vi "8P_EnFlo_Specific.vi"(4 "Datalog file path (full)":path, 5 "COM port":refnum<visa-resource-name>, 6 "Log data stream":bool, 7 "Data rate (Hz)":u8(ring)=14 items=["1", "2", "4", "5", "8", "10", "16", "20", "25", "32", "40", "50", "64", "80", "100", "125", "160", "200", "250", "320", "400", "500", "625", "800", "1000"], 8 "N samples":u32=1000, 9 "Command":T2="s") -> (0 "Output Freq Hz":dbl, 1 "Error":errorcluster, 2 "All samples out":sgl[][](array[numeric]), 3 "Rendezvous Out":bool)   [LabVIEW 2020]
uses:
  ctls/Cmd.ctl
  <vilib>/Analysis/baseanly.llb/Mean (DBL).vi
  <vilib>/Analysis/NI_AALBase.lvlib
  Globals/Meas_global.vi
panel:
  in  "Main":T1(tab)
  out "Pressure sensor EEPROM checksums ok":bool[](array[boolean])
  out "Pressure sensor temperatures in range":bool[](array[boolean])
  out "Pressure sensor values in range":bool[](array[boolean])
  out "Subsystems ok":bool[](array[boolean])
  out "P_raw_Azero":sgl[](array[numeric])
  out "n":u16
  out "Auto zero progBar":u16(slide) caption="Collecting samples, please maintain dP = 0" scale=0.0..1000.0
  out "Chk ok":bool
  out "EEPROM Checksum":u8 format="%02x"
  in  "EEPROM array":sgl[](array[numeric])
  out "No of Samples Requested":u32
  out "No of Samples Acquired":i32
  out "Downsampling (N)":i32
  out "Acquisiton Freq Hz":dbl
  out "sent":bool
  in  "Stop Data":bool
  out "External thermistor temperature (°C)":sgl
  out "Checksum ok":bool
  out "Pressures":sgl[][](graph)
  out "Stream enabled":bool
  out "frm err":u32
  out "chk err":u32
  # "Paul Nathan 08/2017"
  # "Output array order:\nP0......... (Pa)\n.\n.\nP7......... (Pa)\nT_ext.... (deg C)\nT0..........(deg C)\n.\n.\nT7......... (deg C)"
  # "External thermistor value in range"
  # "MCU EEPROM checksum ok"
  # "Pressure sensor 0 EEPROM checksum okay"
  # "Pressure sensor 1 EEPROM checksum okay"
  # "Pressure sensor 2 EEPROM checksum okay"
  # "Pressure sensor 3 EEPROM checksum okay"
  # "Pressure sensor 4 EEPROM checksum okay"
  # "Pressure sensor 5 EEPROM checksum okay"
  # "Pressure sensor 6 EEPROM checksum okay"
  # "Pressure sensor 0 temperature in range"
  # "Pressure sensor 1 temperature in range"
  # "Pressure sensor 2 temperature in range"
  # "Pressure sensor 3 temperature in range"
  # "Pressure sensor 4 temperature in range"
  # "Pressure sensor 5 temperature in range"
  # "Pressure sensor 6 temperature in range"
  # "Pressure sensor 0 value in range"
  # "Pressure sensor 1 value in range"
  # "Pressure sensor 2 value in range"
  # "Pressure sensor 3 value in range"
  # "Pressure sensor 4 value in range"
  # "Pressure sensor 5 value in range"
  # "Pressure sensor 6 value in range"
  # "of 1000"
  # "P0 raw auto-zero"
  # "P1 raw auto-zero"
  # "P2 raw auto-zero"
  # "P3 raw auto-zero"
  # "P4 raw auto-zero"
  # "P5 raw auto-zero"
  # "P6 raw auto-zero"
  # "P7 raw auto-zero"
  # "P0 raw auto-zero"
  # "P1 raw auto-zero"
  # "P2 raw auto-zero"
  # "P3 raw auto-zero"
  # "P4 raw auto-zero"
  # "P5 raw auto-zero"
  # "P6 raw auto-zero"
  # "P7 raw auto-zero"
  # "External thermistor temperature offset (deg C)"
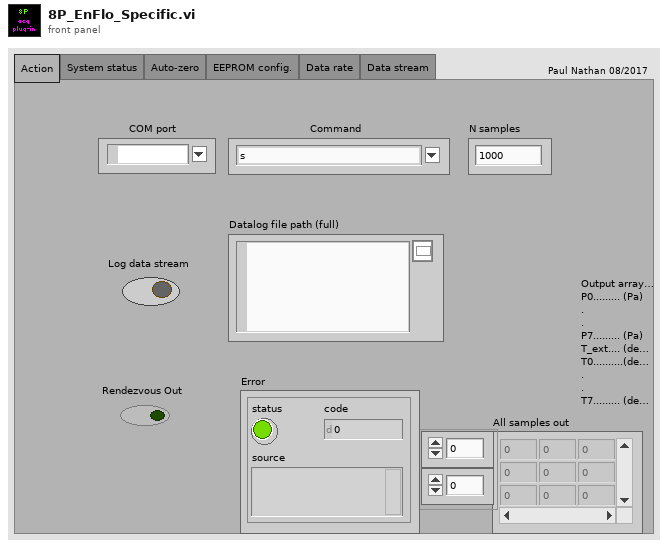
[diagram p1: front panel]
types:
  T1 = enum32{"Action", "System status", "Auto-zero", "EEPROM config.", "Data rate", "Data stream"}
  T2 = typedef "Cmd.ctl" = string
  T3 = enum16{"open", "replace", "create", "open or create", "replace or create", "replace or create with confirmation"}
  T4 = typedef "Rendezvous RefNum" = refnum<k1>
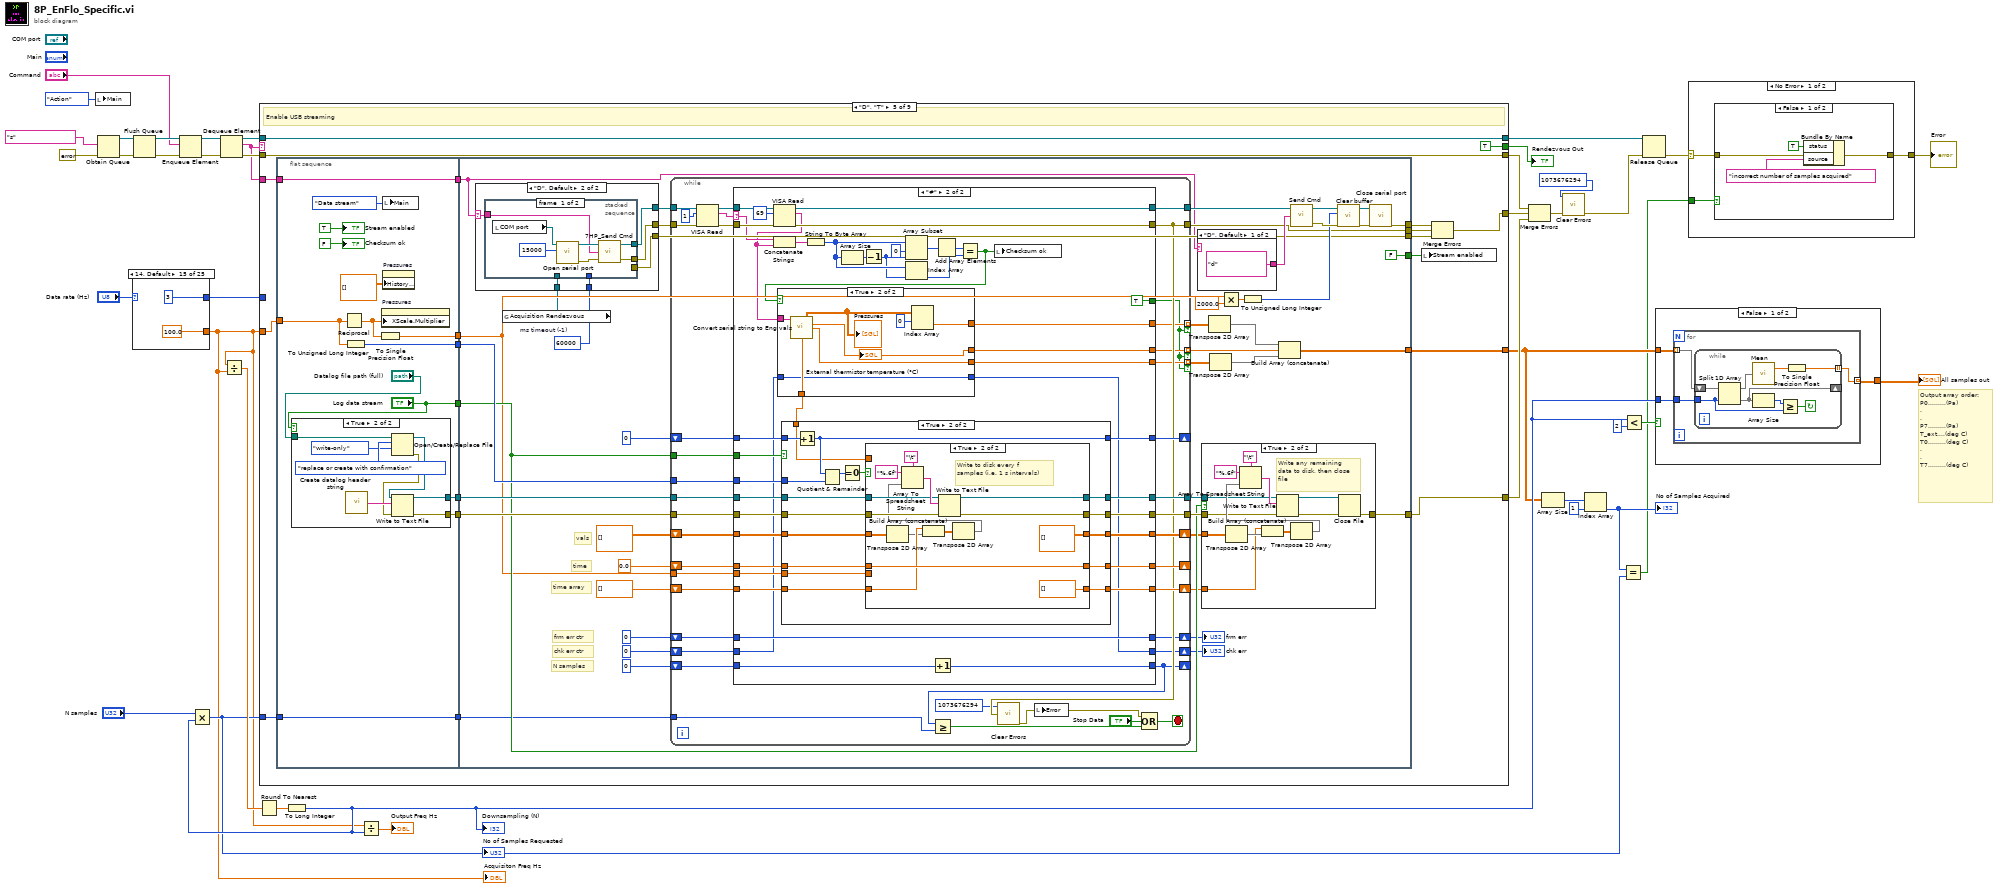
[diagram p0: block diagram]
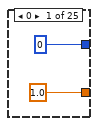
[diagram p5: hidden frame]
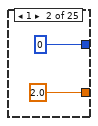
[diagram p6: hidden frame]
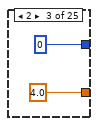
[diagram p7: hidden frame]
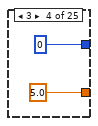
[diagram p8: hidden frame]
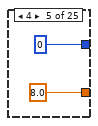
[diagram p9: hidden frame]
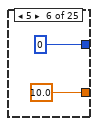
[diagram p10: hidden frame]
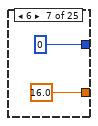
[diagram p11: hidden frame]
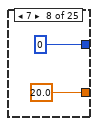
[diagram p12: hidden frame]
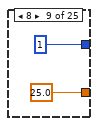
[diagram p13: hidden frame]
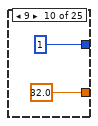
[diagram p14: hidden frame]
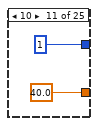
[diagram p15: hidden frame]
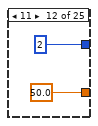
[diagram p16: hidden frame]
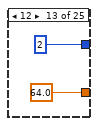
[diagram p17: hidden frame]
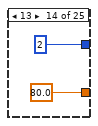
[diagram p18: hidden frame]
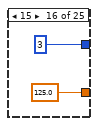
[diagram p19: hidden frame]
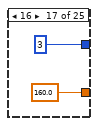
[diagram p20: hidden frame]
diagram:
  # "Output array order:\nP0.........(Pa)\n.\n.\nP7.........(Pa)\nT_ext....(deg C)\nT0.........(deg C)\n.\n.\nT7.........(deg C)"
  n1 = local write "Main"(T1."Action" ("Main")) -> ()
  n2 = Obtain Queue(element data type=T2 "s" ("Combo Box"), error in (no error)=errorcluster {"status"=FALSE, "code"=0, "source"=""}) -> (queue out=w38:refnum<queue>, error out=w39:errorcluster)  [unwired: 3 in, 1 out]
  n3 = case shown="14, Default" "Data rate (Hz)" {
    tunnel: [1.0 2.0 4.0 5.0 8.0 10.0 16.0 20.0 25.0 32.0 40.0 50.0 64.0 80.0 100.0 125.0 160.0 200.0 250.0 320.0 400.0 500.0 625.0 800.0 1000.0] -> w2
    tunnel: [u8 0 u8 0 u8 0 u8 0 u8 0 u8 0 u8 0 u8 0 u8 1 u8 1 u8 1 u8 2 u8 2 u8 2 u8 3 u8 3 u8 3 u8 4 u8 4 u8 4 u8 5 u8 5 u8 6 u8 6 u8 6] -> w1
    frame 0 {
    }
    frame 1 {
    }
    frame 2 {
    }
    frame 3 {
    }
    frame 4 {
    }
    frame 5 {
    }
    frame 6 {
    }
    frame 7 {
    }
    frame 8 {
    }
    frame 9 {
    }
    frame 10 {
    }
    frame 11 {
    }
    frame 12 {
    }
    frame 13 {
    }
    frame 14, Default {
    }
    frame 15 {
    }
    frame 16 {
    }
    frame 17 {
    }
    frame 18 {
    }
    frame 19 {
    }
    frame 20 {
    }
    frame 21 {
    }
    frame 22 {
    }
    frame 23 {
    }
    frame 24 {
    }
  }
  "Acquisiton Freq Hz" <- w2
  n4 = Flush Queue(queue=w38, error in (no error)=w39) -> (queue out=w37:refnum<queue>, error out=w33:errorcluster)  [unwired: 1 out]
  n5 = Enqueue Element(queue=w37, element="Command", error in (no error)=w33) -> (queue out=w34:refnum<queue>, error out=w32:errorcluster)  [unwired: 1 in, 1 out]
  n6 = Dequeue Element(queue=w34, error in (no error)=w32) -> (queue out=w29:refnum<queue>, element=w27:T2, error out=w28:errorcluster)  [unwired: 1 in, 1 out]
  n7 = Divide(x=w2, y=w2) -> (x/y=w17:dbl)
  n8 = Round To Nearest(number=w17) -> (nearest integer value=w16:dbl)
  n9 = To Long Integer(number=w16) -> (32bit integer=w12:i32)
  "Downsampling (N)" <- w12
  n10 = Multiply(x="N samples", y=w12) -> (x*y=w4:u32)
  "No of Samples Requested" <- w4
  n11 = case shown="\"D\", \"T\"" w27 {
    tunnel: w29 -> [w96 w135 w172 w213 w265 w544 w574 w601 w605]
    tunnel: [w96 w135 w172 w213 w265 w544 w574 w601 w605] -> w30
    tunnel: w28 -> [w95 w134 w171 w212 w264 w543 w575 w600 w604]
    tunnel: [w95 w134 w171 w212 w264 w543 w575 w600 w604] -> w26
    tunnel: w27 -> [w94 w133 w170 w211 w263 w546 w572 _ _]
    tunnel: [w92 w131 w168 w208 w248 w545 w570 errorcluster {"status"=FALSE, "code"=0, "source"=""} ("Error out") errorcluster {"status"=FALSE, "code"=0, "source"=""} ("Error out")] -> w25
    tunnel: [_ _ _ _ w261 _ _ _ _] -> w24
    tunnel: w2 -> [_ _ _ _ w257 w542 w568 _ _]
    tunnel: w4 -> [_ _ _ _ w253 _ _ _ _]
    tunnel: [_ _ _ _ w251 _ _ _ _] -> w11
    tunnel: [FALSE FALSE FALSE FALSE TRUE FALSE FALSE FALSE FALSE] -> w3
    tunnel: w1 -> [_ _ _ _ _ _ w567 _ _]
    frame "S", "s" {
      # "Perform self-test and retrieve status bytes, Retrieve status bytes"
      n12 = flat-sequence {
        tunnel: w94 -> [w99]
        tunnel: [w99] -> w93
        tunnel: w93 -> [w105]
        tunnel: [w100] -> w92
        frame #0 {
          w98 = bool[] [] ("Pressure sensor EEPROM checksums ok")
          n13 = local write "Main"(T1."System status" ("Main")) -> ()
          "Pressure sensor EEPROM checksums ok" <- w98
          "Pressure sensor temperatures in range" <- w98
          "Pressure sensor values in range" <- w98
          "Subsystems ok" <- w98
        }
        frame #1 {
          w109 = 1 ("length (rest)")
          w117 = u8 0 ("byte count")
          n14 = local read "COM port"() -> (w106:refnum<visa-resource-name>)
          n15 = call "Open serial port.vi"("timeout (ms)"=u32 5000, "VISA resource name"=w106) -> ("Error out"=w127:errorcluster, "VISA resource name out"=w128:refnum<visa-resource-name>)  [unwired: 8 in]
          n16 = call "Send Cmd.vi"("Error In"=w127, "Operation"=w105, "Port"=w128) -> ("Error Out"=w125:errorcluster, "Port out"=w126:refnum<visa-resource-name>)  [unwired: 1 in]
          n17 = VISA Read(VISA resource name=w126, byte count=u32 4, error in (no error)=w125) -> (VISA resource name out=w123:refnum<visa-resource-name>, read buffer=w112:string, error out=w122:errorcluster)  [unwired: 1 out]
          n18 = call "Close serial port.vi"("Error in"=w122, "VISA resource name"=w123) -> ("Error out"=w100:errorcluster)  [unwired: 9 in]
          n19 = String Subset(string=w112, offset (0)=0, length (rest)=w109) -> (substring=w121:string)
          n20 = String Subset(string=w112, offset (0)=1, length (rest)=w109) -> (substring=w120:string)
          n21 = String Subset(string=w112, offset (0)=2 ("length (rest)"), length (rest)=w109) -> (substring=w119:string)
          n22 = String Subset(string=w112, offset (0)=3, length (rest)=w109) -> (substring=w118:string)
          n23 = Type Cast(type=w117, x=w121) -> (*(type *) &x=w116:u8)
          n24 = Type Cast(type=w117, x=w120) -> (*(type *) &x=w115:u8)
          n25 = Type Cast(type=w117, x=w119) -> (*(type *) &x=w114:u8)
          n26 = Type Cast(type=w117, x=w118) -> (*(type *) &x=w113:u8)
          n27 = Number To Boolean Array(number=w116) -> (Boolean array=w104:bool[])
          n28 = Number To Boolean Array(number=w115) -> (Boolean array=w103:bool[])
          n29 = Number To Boolean Array(number=w114) -> (Boolean array=w102:bool[])
          n30 = Number To Boolean Array(number=w113) -> (Boolean array=w101:bool[])
          n31 = local write "Pressure sensor EEPROM checksums ok"(w104) -> ()
          n32 = local write "Pressure sensor temperatures in range"(w103) -> ()
          n33 = local write "Pressure sensor values in range"(w102) -> ()
          n34 = local write "Subsystems ok"(w101) -> ()
        }
      }
    }
    frame "Z", "z" {
      # "Perform permanent auto-zero (write values to EEPROM), Perform temporary auto-zero"
      n35 = flat-sequence {
        tunnel: w133 -> [w139]
        tunnel: [w139] -> w132
        tunnel: w132 -> [w146]
        tunnel: [w142] -> w131
        frame #0 {
          n36 = local write "Main"(T1."Auto-zero" ("Main")) -> ()
          "P_raw_Azero" <- sgl[] [] ("P_raw_Azero")
          "Auto zero progBar" <- u16 0 ("Collecting samples, please maintain dP = 0")
        }
        frame #1 {
          n37 = local read "COM port"() -> (w147:refnum<visa-resource-name>)
          n38 = call "Open serial port.vi"("timeout (ms)"=u32 16000, "VISA resource name"=w147) -> ("Error out"=w153:errorcluster, "VISA resource name out"=w154:refnum<visa-resource-name>)  [unwired: 8 in]
          n39 = call "Send Cmd.vi"("Error In"=w153, "Operation"=w146, "Port"=w154) -> ("Error Out"=w151:errorcluster, "Port out"=w152:refnum<visa-resource-name>)  [unwired: 1 in]
          n40 = VISA Read(VISA resource name=w152, byte count=u32 32, error in (no error)=w151) -> (VISA resource name out=w149:refnum<visa-resource-name>, read buffer=w143:string, error out=w148:errorcluster)  [unwired: 1 out]
          n41 = for {
            N: 1000 -> [_]
            shift-right: [w156] -> _
            shift-left: u16 0 -> [w157]
            n42 = Increment(x=w157) -> (x+1=w156:u16)
            "n" <- w156
            n43 = Wait (ms)(milliseconds to wait=u32 11) -> ()  [unwired: 1 out]
            n44 = local write "Auto zero progBar"(w156) -> ()
          }
          n45 = for {
            N: 8 -> [_]
            tunnel: [w160] -> w145 mode=indexing
            tunnel: w143 -> [w159]
            i -> [w166]
            w164 = 4 ("x")
            # "to BE"
            n46 = Multiply(x=w164, y=w166) -> (x*y=w165:i32)
            n47 = String Subset(string=w159, offset (0)=w165, length (rest)=w164) -> (substring=w163:string)
            n48 = Reverse String(1:w163) -> (0:w162:string)
            n49 = Type Cast(type=sgl 0.0 ("byte count"), x=w162) -> (*(type *) &x=w160:sgl)
          }
          n50 = call "Close serial port.vi"("Error in"=w148, "VISA resource name"=w149) -> ("Error out"=w142:errorcluster)  [unwired: 9 in]
          n51 = local write "P_raw_Azero"(w145) -> ()
        }
      }
    }
    frame "R" {
      # "Read all EEPROM values"
      n52 = flat-sequence {
        tunnel: w170 -> [w175]
        tunnel: [w175] -> w169
        tunnel: w169 -> [w189]
        tunnel: [w176] -> w168
        frame #0 {
          n53 = local write "EEPROM array"(sgl[] [] ("EEPROM array")) -> ()
          n54 = local write "Main"(T1."EEPROM config." ("Main")) -> ()
        }
        frame #1 {
          n55 = local read "COM port"() -> (w190:refnum<visa-resource-name>)
          n56 = call "Open serial port.vi"("timeout (ms)"=u32 5000, "VISA resource name"=w190) -> ("Error out"=w196:errorcluster, "VISA resource name out"=w197:refnum<visa-resource-name>)  [unwired: 8 in]
          n57 = call "Send Cmd.vi"("Error In"=w196, "Operation"=w189, "Port"=w197) -> ("Error Out"=w194:errorcluster, "Port out"=w195:refnum<visa-resource-name>)  [unwired: 1 in]
          n58 = VISA Read(VISA resource name=w195, byte count=u32 37, error in (no error)=w194) -> (VISA resource name out=w192:refnum<visa-resource-name>, read buffer=w185:string, error out=w191:errorcluster)  [unwired: 1 out]
          n59 = String To Byte Array(string=w185) -> (unsigned byte array=w179:u8[])
          n60 = call "Close serial port.vi"("Error in"=w191, "VISA resource name"=w192) -> ("Error out"=w176:errorcluster)  [unwired: 9 in]
          n61 = for {
            N: 9 -> [_]
            tunnel: [w202] -> w187 mode=indexing
            tunnel: w185 -> [w201]
            i -> [w206]
            w204 = 4 ("x")
            # "to BE"
            n62 = Multiply(x=w204, y=w206) -> (x*y=w205:i32)
            n63 = String Subset(string=w201, offset (0)=w205, length (rest)=w204) -> (substring=w200:string)
            n64 = Reverse String(1:w200) -> (0:w199:string)
            n65 = Type Cast(type=sgl 0.0 ("byte count"), x=w199) -> (*(type *) &x=w202:sgl)
          }
          n66 = Array Size(array=w179) -> (size(s)=w181:i32)
          n67 = Decrement(x=w181) -> (x-1=w180:i32)
          n68 = Index Array(array=w179, index=36) -> (element=w183:u8)
          n69 = Array Subset(array=w179, index=0, length=w180) -> (w177:u8[])
          n70 = Add Array Elements(numeric array=w177) -> (sum=w178:u8)
          n71 = Equal?(x=w183, y=w178) -> (x = y?=w186:bool)
          n72 = local write "EEPROM array"(w187) -> ()
          n73 = local write "EEPROM Checksum"(w183) -> ()
          n74 = local write "Chk ok"(w186) -> ()
        }
      }
    }
    frame "W" {
      # "Write all EEPROM values (including new checksum)"
      n75 = flat-sequence {
        tunnel: w211 -> [w216]
        tunnel: [w216] -> w210
        tunnel: ["EEPROM array"] -> w209
        tunnel: w210 -> [w231]
        tunnel: w209 -> [w224]
        tunnel: [w217] -> w208
        frame #0 {
          n76 = local write "Main"(T1."EEPROM config." ("Main")) -> ()
        }
        frame #1 {
          n77 = local read "COM port"() -> (w232:refnum<visa-resource-name>)
          n78 = call "Open serial port.vi"("timeout (ms)"=u32 5000, "VISA resource name"=w232) -> ("Error out"=w237:errorcluster, "VISA resource name out"=w238:refnum<visa-resource-name>)  [unwired: 8 in]
          n79 = call "Send Cmd.vi"("Error In"=w237, "Operation"=w231, "Port"=w238) -> ("Error Out"=w235:errorcluster, "Port out"=w236:refnum<visa-resource-name>)  [unwired: 1 in]
          n80 = for {
            N: 9 -> [_]
            tunnel: w224 -> [w242] mode=indexing
            shift-right: [w243] -> w219
            shift-left: "" -> [w244]
            # "to LE"
            n81 = Type Cast(type="", x=w242) -> (*(type *) &x=w241:string)
            n82 = Reverse String(1:w241) -> (0:w240:string)
            n83 = Concatenate Strings(w244, w240) -> (w243:string)
          }
          n84 = String To Byte Array(string=w219) -> (unsigned byte array=w222:u8[])
          n85 = Array Size(array=w222) -> (size(s)=w220:i32)
          n86 = Array Subset(array=w222, index=0, length=w220) -> (w221:u8[])
          n87 = Add Array Elements(numeric array=w221) -> (sum=w218:u8)
          "EEPROM Checksum" <- w218
          n88 = Type Cast(type="", x=w218) -> (*(type *) &x=w227:string)
          n89 = Concatenate Strings(w219, w227) -> (w226:string)
          n90 = VISA Write(VISA resource name=w236, write buffer=w226, error in (no error)=w235) -> (VISA resource name out=w234:refnum<visa-resource-name>, error out=w233:errorcluster)  [unwired: 1 out]
          n91 = call "Close serial port.vi"("Error in"=w233, "VISA resource name"=w234) -> ("Error out"=w217:errorcluster)  [unwired: 9 in]
          "Chk ok" <- TRUE ("Chk ok")
        }
      }
    }
    frame "D", "T" {
      # "Enable USB streaming"
      n92 = flat-sequence {
        tunnel: w263 -> [w279]
        tunnel: [w279] -> w262
        tunnel: [w276] -> w260
        tunnel: [w275] -> w259
        tunnel: [w273] -> w258
        tunnel: w257 -> [w274]
        tunnel: [w271] -> w256
        tunnel: ["Log data stream"] -> w255
        tunnel: w253 -> [w267]
        tunnel: [w267] -> w252
        tunnel: w262 -> [w292]
        tunnel: [w333] -> w249
        tunnel: [w332] -> w261
        tunnel: w260 -> [w329]
        tunnel: w259 -> [w328]
        tunnel: w258 -> [w330]
        tunnel: w256 -> [w314]
        tunnel: w255 -> [w322]
        tunnel: [FALSE] -> w254
        tunnel: w252 -> [w308]
        tunnel: [w305] -> w251
        tunnel: [w294] -> w247
        tunnel: [w293] -> w246
        frame #0 {
          n93 = case shown="True" "Log data stream" {
            tunnel: "Datalog file path (full)" -> [_ w289]
            tunnel: [refnum<file> refnum ("refnum out") w283] -> w276
            tunnel: [errorcluster {"status"=FALSE, "code"=0, "source"=""} ("error out") w282] -> w275
            frame False {
            }
            frame True {
              n94 = call "Create datalog header string.vi"() -> ("Datalog header string"=w285:string)  [unwired: 1 in]
              n95 = Open/Create/Replace File(file path (use dialog)=w289, operation (0:open)=T3."replace or create with confirmation", access (0:read/write)=enum16{"read/write", "read-only", "write-only"}."write-only") -> (refnum out=w286:refnum<file>, error out=w284:errorcluster)  [unwired: 3 in, 1 out]
              n96 = Write to Text File(file (use dialog)=w286, text=w285, error in=w284) -> (refnum out=w283:refnum<file>, error out=w282:errorcluster)  [unwired: 1 in, 1 out]
            }
          }
          n97 = Reciprocal(x=w274) -> (1/x=w272:dbl)
          n98 = To Unsigned Long Integer(number=w274) -> (unsigned 32bit integer=w273:u32)
          n99 = To Single Precision Float(number=w272) -> (single precision float=w271:sgl)
          n100 = property on="Pressures" class="WFChart (strict)"("XScale.Multiplier"=w272) -> ()  [unwired: 2 in, 2 out]
          n101 = local write "Main"(T1."Data stream" ("Main")) -> ()
          n102 = property on="Pressures" class="WFChart (strict)"("History Data"=sgl[][] []) -> ()  [unwired: 2 in, 2 out]
          "Checksum ok" <- FALSE ("Checksum ok")
          "Stream enabled" <- TRUE ("Stream enabled")
        }
        frame #1 {
          w298 = 60000  # ms timeout (-1)
          # "N samples"
          # "chk err ctr"
          # "frm err ctr"
          # "vals"
          # "time"
          # "time array"
          n103 = global read "Meas_global.vi" "Acquisition Rendezvous"() -> (w297:T4)
          n104 = case shown="\"D\", Default" w292 {
            selector: w292 -> [w339 w355]
            tunnel: [w338 w354] -> w295
            tunnel: [w337 w353] -> w296
            tunnel: [w336 w352] -> w293
            tunnel: w297 -> [w335 w351]
            tunnel: w298 -> [w334 w350]
            frame "T" {
              n105 = stacked-sequence {
                tunnel: w339 -> [w342 _]
                tunnel: [w341 _] -> w338
                tunnel: [w340 _] -> w337
                tunnel: [_ w349] -> w336
                tunnel: w335 -> [_ w348]
                tunnel: w334 -> [_ w347]
                frame #0 {
                  n106 = local read "COM port"() -> (w343:refnum<visa-resource-name>)
                  n107 = call "Open serial port.vi"("timeout (ms)"=u32 15000, "VISA resource name"=w343) -> ("Error out"=w346:errorcluster, "VISA resource name out"=w345:refnum<visa-resource-name>)  [unwired: 8 in]
                  n108 = call "7HP_Send Cmd, wait for ack.vi"("Error In"=w346, "Operation"=w342, "Port"=w345) -> ("Error Out"=w341:errorcluster, "Port out"=w340:refnum<visa-resource-name>)  [unwired: 1 out]
                }
                frame #1 {
                  # "Wait here until all acq. devs. are ready."
                  n109 = call <vilib>:"Wait at Rendezvous.vi"("ms timeout (-1)"=w347, "rendezvous"=w348) -> ("error out"=w349:errorcluster)  [unwired: 3 in, 2 out]
                }
              }
            }
            frame "D", Default {
              n110 = stacked-sequence {
                tunnel: w355 -> [w359 _]
                tunnel: [w356 _] -> w354
                tunnel: [w357 _] -> w353
                tunnel: [_ w365] -> w352
                tunnel: w351 -> [_ w364]
                tunnel: w350 -> [_ w363]
                frame #0 {
                  n111 = local read "COM port"() -> (w361:refnum<visa-resource-name>)
                  n112 = call "Open serial port.vi"("timeout (ms)"=u32 15000, "VISA resource name"=w361) -> ("Error out"=w358:errorcluster, "VISA resource name out"=w360:refnum<visa-resource-name>)  [unwired: 8 in]
                  n113 = call "7HP_Send Cmd.vi"("Error In"=w358, "Operation"=w359, "Port"=w360) -> ("Error Out"=w356:errorcluster, "Port out"=w357:refnum<visa-resource-name>)  [unwired: 1 in]
                }
                frame #1 {
                  # "Wait here until all acq. devs. are ready."
                  n114 = call <vilib>:"Wait at Rendezvous.vi"("ms timeout (-1)"=w363, "rendezvous"=w364) -> ("error out"=w365:errorcluster)  [unwired: 3 in, 2 out]
                }
              }
            }
          }
          n115 = while {
            tunnel: [w396] -> w294
            tunnel: w296 -> [w398]
            tunnel: [w416] -> w321
            shift-right: [w412] -> _
            shift-left: u32 0 -> [w413]
            tunnel: w330 -> [w411]
            tunnel: w329 -> [w410]
            tunnel: w328 -> [w409]
            tunnel: [w408] -> w327
            tunnel: [w407] -> w326
            shift-right: [w406] -> w311
            shift-left: sgl[][] [] -> [w405]
            shift-right: [w402] -> _
            shift-left: sgl 0.0 ("Numeric") -> [w404]
            tunnel: w314 -> [w403]
            shift-right: [w400] -> w310
            shift-left: sgl[] [] -> [w401]
            tunnel: w322 -> [w399]
            tunnel: w295 -> [w397]
            shift-right: [w390] -> _
            shift-left: u32 0 -> [w393]
            tunnel: w308 -> [w392]
            tunnel: [w389] -> w307 mode=indexing if=w386
            tunnel: [w388] -> w304 mode=indexing if=w386
            tunnel: [w387] -> w303 mode=indexing if=w386
            shift-right: [w384] -> w291
            shift-left: u32 0 -> [w385]
            shift-right: [w383] -> w290
            shift-left: u32 0 -> [w382]
            stop <- w414 stop-if-true
            n116 = VISA Read(VISA resource name=w398, byte count=u32 1, error in (no error)=w397) -> (VISA resource name out=w418:refnum<visa-resource-name>, read buffer=w419:string, error out=w417:errorcluster)  [unwired: 1 out]
            n117 = case shown="\"#\"" w419 {
              selector: w419 -> [_ w469]
              tunnel: w418 -> [w432 w473]
              tunnel: [w433 w471] -> w396
              tunnel: w417 -> [w433 w474]
              tunnel: [w432 w472] -> w416
              tunnel: w413 -> [w431 w459]
              tunnel: [w431 w458] -> w412
              tunnel: w411 -> [_ w457]
              tunnel: w410 -> [w430 w456]
              tunnel: w409 -> [w429 w455]
              tunnel: [w429 w454] -> w408
              tunnel: [w430 w453] -> w407
              tunnel: [w428 w452] -> w406
              tunnel: w405 -> [w428 w451]
              tunnel: w404 -> [w427 w450]
              tunnel: w403 -> [_ w449]
              tunnel: [w427 w448] -> w402
              tunnel: w401 -> [w426 w447]
              tunnel: [w426 w446] -> w400
              tunnel: w399 -> [_ w445]
              tunnel: w393 -> [w425 w436]
              tunnel: [w425 w444] -> w390
              tunnel: [_ w443] -> w389
              tunnel: [FALSE TRUE] -> w386
              tunnel: [_ w441] -> w388
              tunnel: [_ w440] -> w387
              tunnel: w385 -> [w423 w438]
              tunnel: [w422 w438] -> w384
              tunnel: [w421 w434] -> w383
              tunnel: w382 -> [w421 w435]
              frame Default {
                n118 = Increment(x=w423) -> (x+1=w422:u32)
              }
              frame "#" {
                n119 = VISA Read(VISA resource name=w473, byte count=u32 69, error in (no error)=w474) -> (VISA resource name out=w472:refnum<visa-resource-name>, read buffer=w460:string, error out=w471:errorcluster)  [unwired: 1 out]
                n120 = Concatenate Strings(w469, w460) -> (w461:string)
                n121 = String To Byte Array(string=w461) -> (unsigned byte array=w464:u8[])
                n122 = Array Size(array=w464) -> (size(s)=w467:i32)
                n123 = Decrement(x=w467) -> (x-1=w463:i32)
                n124 = Array Subset(array=w464, index=0, length=w463) -> (w468:u8[])
                n125 = Index Array(array=w464, index=w463) -> (element=w462:u8)
                n126 = Increment(x=w436) -> (x+1=w444:u32)
                n127 = Add Array Elements(numeric array=w468) -> (sum=w465:u8)
                n128 = Equal?(x=w465, y=w462) -> (x = y?=w437:bool)
                n129 = case shown="True" w437 {
                  tunnel: w460 -> [_ w491]
                  tunnel: [w480 w484] -> w443
                  tunnel: [sgl nan ("element") w490] -> w441
                  tunnel: [w480 w489] -> w440
                  tunnel: [w478 w488] -> w439
                  tunnel: w435 -> [w482 w485]
                  tunnel: [w481 w485] -> w434
                  frame False {
                    n130 = Initialize Array(sgl nan ("element"), 8 ("dimension size")) -> (w480:sgl[])
                    n131 = Initialize Array(sgl nan ("element"), 17 ("dimension size")) -> (w478:sgl[])
                    n132 = Increment(x=w482) -> (x+1=w481:u32)
                  }
                  frame True {
                    n133 = call "Convert serial string to Eng vals.vi"("Serial buffer string (excluding FrameChar)"=w491) -> ("Pressures"=w487:sgl[][], "External thermistor temperature (deg C)"=w490:sgl, "Sensor die temperatures (deg C)"=w489:sgl[], "All vals"=w488:sgl[])  [unwired: 11 in]
                    "Pressures" <- w487
                    "External thermistor temperature (°C)" <- w490
                    n134 = Index Array(array=w487, index (row)=0) -> (element=w484:sgl[])  [unwired: 1 in]
                  }
                }
                n135 = case shown="True" w445 {
                  tunnel: w459 -> [w497 w514]
                  tunnel: [w497 w513] -> w458
                  tunnel: w457 -> [_ w512]
                  tunnel: w439 -> [_ w509]
                  tunnel: w456 -> [w495 w508]
                  tunnel: w455 -> [w496 w507]
                  tunnel: [w496 w506] -> w454
                  tunnel: [w495 w505] -> w453
                  tunnel: w451 -> [w494 w504]
                  tunnel: [w494 w503] -> w452
                  tunnel: w450 -> [w493 w502]
                  tunnel: w449 -> [_ w501]
                  tunnel: [w493 w500] -> w448
                  tunnel: w447 -> [w492 w499]
                  tunnel: [w492 w498] -> w446
                  frame False {
                  }
                  frame True {
                    n136 = Increment(x=w514) -> (x+1=w513:u32)
                    n137 = Quotient & Remainder(x=w513, y=w512) -> (x-y*floor(x/y)=w511:u32)  [unwired: 1 out]
                    n138 = Equal To 0?(x=w511) -> (x = 0?=w510:bool)
                    n139 = case shown="True" w510 {
                      tunnel: w509 -> [w522 _]
                      tunnel: w508 -> [w523 w536]
                      tunnel: w507 -> [w524 w535]
                      tunnel: [w524 w534] -> w506
                      tunnel: [w523 w533] -> w505
                      tunnel: w504 -> [w516 w528]
                      tunnel: [w515 sgl[][] []] -> w503
                      tunnel: w502 -> [w517 w531]
                      tunnel: w501 -> [w521 _]
                      tunnel: [w520 w531] -> w500
                      tunnel: w499 -> [w519 w530]
                      tunnel: [w518 sgl[] []] -> w498
                      frame False {
                        n140 = Add(x=w517, y=w521) -> (x+y=w520:sgl)
                        n141 = Build Array (concatenate)(w516, w522) -> (w515:sgl[][])
                        n142 = Build Array (concatenate)(w519, w517) -> (w518:sgl[])
                      }
                      frame True {
                        # "Write to disk every f samples (i.e. 1 s intervals)"
                        n143 = Transpose 2D Array(2D array=w528) -> (transposed array=w527:sgl[][])
                        n144 = Build Array (concatenate)(w530, w527) -> (w526:sgl[][])
                        n145 = Transpose 2D Array(2D array=w526) -> (transposed array=w525:sgl[][])
                        n146 = Array To Spreadsheet String(delimiter (Tab)="\t", array=w525, 3:"%.6f" ("format string")) -> (spreadsheet string=w539:string)
                        n147 = Write to Text File(file (use dialog)=w536, text=w539, error in=w535) -> (refnum out=w533:refnum<file>, error out=w534:errorcluster)  [unwired: 1 in, 1 out]
                      }
                    }
                  }
                }
                n148 = local write "Checksum ok"(w437) -> ()
              }
            }
            n149 = Greater Or Equal?(x=w390, y=w392) -> (x >= y?=w391:bool)
            n150 = call <vilib>:"Clear Errors.vi"("error in (no error)"=w396, "specific error code to clear (0: all)"=1073676294) -> ("error out"=w395:errorcluster)  [unwired: 4 in, 1 out]
            n151 = local write "Error"(w395) -> ()
            n152 = Compound Arithmetic op=OR(w395, "Stop Data", w391) -> (w414:bool)
          }
          "frm err" <- w291
          "chk err" <- w290
          n153 = case shown="\"D\", Default" w292 {
            tunnel: [T2 "d" ("Combo Box") T2 "t" ("Combo Box")] -> w301
            frame "D", Default {
            }
            frame "T" {
            }
          }
          n154 = case shown="True" w322 {
            tunnel: [w368 w381] -> w332
            tunnel: w327 -> [w368 w373]
            tunnel: w326 -> [_ w374]
            tunnel: w311 -> [_ w372]
            tunnel: w310 -> [_ w371]
            frame False {
            }
            frame True {
              # "Write any remaining data to disk, then close file"
              n155 = Transpose 2D Array(2D array=w372) -> (transposed array=w378:sgl[][])
              n156 = Build Array (concatenate)(w371, w378) -> (w379:sgl[][])
              n157 = Transpose 2D Array(2D array=w379) -> (transposed array=w380:sgl[][])
              n158 = Array To Spreadsheet String(delimiter (Tab)="\t", array=w380, 3:"%.6f" ("format string")) -> (spreadsheet string=w375:string)
              n159 = Write to Text File(file (use dialog)=w374, text=w375, error in=w373) -> (refnum out=w370:refnum<file>, error out=w369:errorcluster)  [unwired: 1 in, 1 out]
              n160 = Close File(refnum=w370, error in=w369) -> (error out=w381:errorcluster)  [unwired: 1 out]
            }
          }
          n161 = Transpose 2D Array(2D array=w307) -> (transposed array=w306:sgl[][])
          n162 = Transpose 2D Array(2D array=w303) -> (transposed array=w302:sgl[][])
          n163 = Multiply(x=w314, y=sgl 2000.0) -> (x*y=w315:sgl)
          n164 = To Unsigned Long Integer(number=w315) -> (unsigned 32bit integer=w312:u32)
          n165 = Build Array (concatenate)(w306, w304, w302) -> (w305:sgl[][])
          n166 = call "Send Cmd.vi"("Operation"=w301, "Port"=w321) -> ("Error Out"=w318:errorcluster, "Port out"=w319:refnum<visa-resource-name>)  [unwired: 2 in]
          n167 = call "Clear buffer.vi"("Error in"=w318, "dt for timeout (ms)"=w312, "VISA resource name in"=w319) -> ("Error out"=w316:errorcluster, "VISA resource name out"=w317:refnum<visa-resource-name>)  [unwired: 3 in]
          n168 = call "Close serial port.vi"("Error in"=w316, "VISA resource name"=w317) -> ("Error out"=w333:errorcluster)  [unwired: 9 in]
        }
      }
      n169 = local write "Stream enabled"(w254) -> ()
      n170 = Merge Errors(w249, w247, w246) -> (w248:errorcluster)
    }
    frame "d", "t" {
      # "Disable USB streaming"
      n171 = flat-sequence {
        tunnel: [w554] -> w547
        tunnel: w546 -> [w554]
        tunnel: w542 -> [w549]
        tunnel: [w548] -> w541
        tunnel: w547 -> [w562]
        tunnel: [w561] -> w545
        tunnel: w541 -> [w556]
        frame #0 {
          n172 = Reciprocal(x=w549) -> (1/x=w551:dbl)
          n173 = disable-structure shown="Disabled" {
            frame Disabled {
              n174 = local write "Main"(T1."Data stream" ("Main")) -> ()
            }
            frame Enabled {
            }
          }
          n175 = To Single Precision Float(number=w551) -> (single precision float=w553:sgl)
          n176 = Multiply(x=w553, y=sgl 2000.0) -> (x*y=w552:sgl)
          n177 = To Unsigned Long Integer(number=w552) -> (unsigned 32bit integer=w548:u32)
        }
        frame #1 {
          n178 = local read "COM port"() -> (w563:refnum<visa-resource-name>)
          n179 = call "Open serial port.vi"("timeout (ms)"=u32 5000, "VISA resource name"=w563) -> ("Error out"=w564:errorcluster, "VISA resource name out"=w565:refnum<visa-resource-name>)  [unwired: 8 in]
          n180 = call "Send Cmd.vi"("Error In"=w564, "Operation"=w562, "Port"=w565) -> ("Error Out"=w560:errorcluster, "Port out"=w558:refnum<visa-resource-name>)  [unwired: 1 in]
          n181 = call "Clear buffer.vi"("Error in"=w560, "dt for timeout (ms)"=w556, "VISA resource name in"=w558) -> ("Error out"=w559:errorcluster, "VISA resource name out"=w557:refnum<visa-resource-name>)  [unwired: 3 in]
          n182 = call "Close serial port.vi"("Error in"=w559, "VISA resource name"=w557) -> ("Error out"=w561:errorcluster)  [unwired: 9 in]
        }
      }
    }
    frame "F" {
      # "Set data rate"
      n183 = flat-sequence {
        tunnel: [w576] -> w573
        tunnel: w572 -> [w576]
        tunnel: w573 -> [w583]
        tunnel: [w582] -> w571
        tunnel: w568 -> [w580]
        tunnel: w567 -> [w579]
        tunnel: w571 -> [w595]
        tunnel: [w595] -> w570
        frame #0 {
          n184 = local write "Main"(T1."Data rate" ("Main")) -> ()
          n185 = local write "sent"(FALSE ("sent")) -> ()
        }
        frame #1 {
          w585 = ""
          # "to LE"
          n186 = local read "COM port"() -> (w581:refnum<visa-resource-name>)
          n187 = To Unsigned Word Integer(number=w580) -> (unsigned 16bit integer=w593:u16)
          n188 = Type Cast(type=w585, x=w579) -> (*(type *) &x=w594:string)
          n189 = Type Cast(type=w585, x=w593) -> (*(type *) &x=w587:string)
          n190 = call "Open serial port.vi"("timeout (ms)"=u32 5000, "VISA resource name"=w581) -> ("Error out"=w591:errorcluster, "VISA resource name out"=w592:refnum<visa-resource-name>)  [unwired: 8 in]
          n191 = Reverse String(1:w587) -> (0:w586:string)
          n192 = Concatenate Strings(w594, w586) -> (w588:string)
          n193 = call "Send Cmd + Data.vi"("Error In"=w591, "Data"=w588, "Operation"=w583, "Port"=w592) -> ("Error Out"=w589:errorcluster, "Port out"=w590:refnum<visa-resource-name>)  [unwired: 1 in]
          n194 = call "Close serial port.vi"("Error in"=w589, "VISA resource name"=w590) -> ("Error out"=w582:errorcluster)  [unwired: 9 in]
        }
        frame #2 {
          n195 = Unbundle By Name(w595) -> ("status"=w597:bool)
          n196 = Not(x=w597) -> (.not. x?=→"sent":bool)
        }
      }
    }
    frame "X" {
      # "Exit"
    }
    frame Default {
    }
  }
  "Rendezvous Out" <- w3
  n197 = Divide(x=w2, y=w12) -> (x/y=→"Output Freq Hz":dbl)
  n198 = Merge Errors(w26, w25, w24) -> (w23:errorcluster)
  n199 = Array Size(array=w11) -> (size(s)=w10:i32[])
  n200 = call <vilib>:"Clear Errors.vi"("error in (no error)"=w23, "specific error code to clear (0: all)"=1073676294) -> ("error out"=w31:errorcluster)  [unwired: 4 in, 1 out]
  n201 = Index Array(array=w10, index=1) -> (element=w8:i32)
  "No of Samples Acquired" <- w8
  n202 = Equal?(x=w8, y=w4) -> (x = y?=w5:bool)
  n203 = Less?(x=w12, y=2) -> (x < y?=w18:bool)
  n204 = Release Queue(queue=w30, error in (no error)=w31) -> (error out=w7:errorcluster)  [unwired: 1 in, 2 out]
  n205 = case shown="False" w18 {
    tunnel: w11 -> [w606 w620]
    tunnel: [w608 w620] -> w15
    tunnel: w12 -> [w607 _]
    frame False {
      n206 = for {
        tunnel: [w611] -> w608 mode=indexing
        tunnel: w607 -> [w610]
        tunnel: w606 -> [w609] mode=indexing
        n207 = while {
          shift-right: [w617] -> _
          shift-left: w609 -> [w619]
          tunnel: w610 -> [w616]
          tunnel: [w612] -> w611 mode=indexing
          stop <- w615 continue-if-true
          n208 = Split 1D Array(array=w619, index=w616) -> (first subarray=w618:sgl[], second subarray=w617:sgl[])
          n209 = call-poly <vilib>:"Mean.vi"("X"=w618) -> ("mean"=w613:dbl)  [unwired: 1 out]
          n210 = Array Size(array=w617) -> (size(s)=w614:i32)
          n211 = Greater Or Equal?(x=w614, y=w616) -> (x >= y?=w615:bool)
          n212 = To Single Precision Float(number=w613) -> (single precision float=w612:sgl)
        }
      }
    }
    frame True {
    }
  }
  "All samples out" <- w15
  n213 = case shown="No Error" w7 {
    selector: w7 -> [w622 w629]
    tunnel: [w621 w629] -> w6
    tunnel: w5 -> [w623 _]
    frame No Error {
      n214 = case shown="False" w623 {
        tunnel: w622 -> [w627 w628]
        tunnel: [w624 w628] -> w621
        frame False {
          n215 = Bundle By Name(cluster=w627, "status"=TRUE, "source"="incorrect number of samples acquired") -> (w624:errorcluster)
        }
        frame True {
        }
      }
    }
    frame Error {
    }
  }
  "Error" <- w6
